vi "Get NG Postion.vi"(8 "error in (no error)":errorcluster, 10 "Current":u16, 11 "Previous":u16) -> (0 "error out":errorcluster, 2 "Station pos":i32[](array[numeric]), 3 "Status":bool)   [LabVIEW 2014]
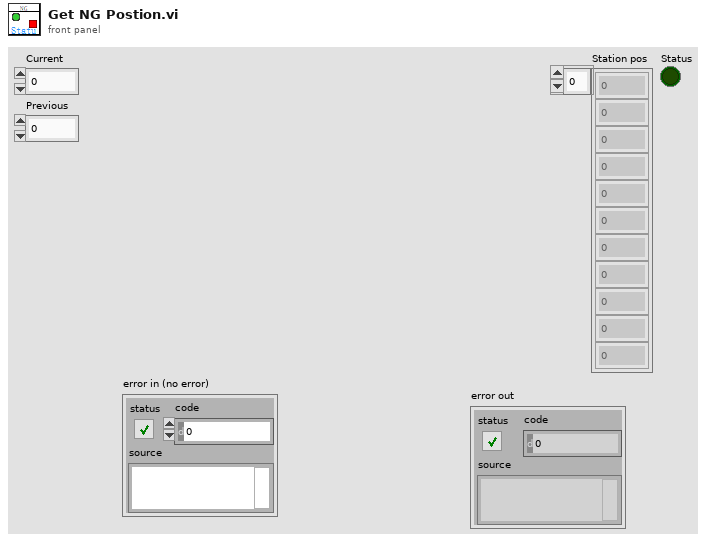
[diagram p1: front panel]
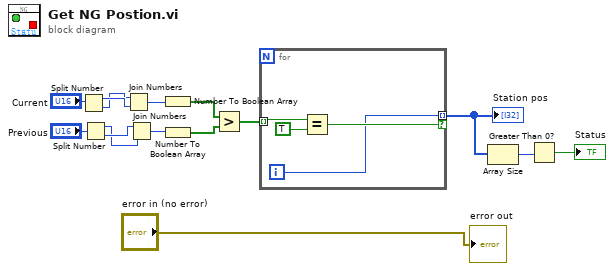
[diagram p0: block diagram]
diagram:
  n1 = Split Number(x="Current") -> (hi(x)=w4:u8, lo(x)=w3:u8)
  n2 = Split Number(x="Previous") -> (hi(x)=w1:u8, lo(x)=w2:u8)
  n3 = Join Numbers(hi=w3, lo=w4) -> ((hi.lo)=w6:u16)
  n4 = Join Numbers(hi=w2, lo=w1) -> ((hi.lo)=w5:u16)
  n5 = Number To Boolean Array(number=w6) -> (Boolean array=w14:bool[])
  n6 = Number To Boolean Array(number=w5) -> (Boolean array=w15:bool[])
  n7 = Greater?(x=w14, y=w15) -> (0:w13:bool[])
  n8 = for {
    tunnel: w13 -> [w19] mode=indexing
    tunnel: [w16] -> w12 mode=indexing if=w17
    i -> [w16]
    n9 = Equal?(x=w19, y=TRUE) -> (x = y?=w17:bool)
  }
  "Station pos" <- w12
  n10 = Array Size(array=w12) -> (size(s)=w11:i32)
  n11 = Greater Than 0?(x=w11) -> (x > 0?=→"Status":bool)
  "error out" <- "error in (no error)"
